vi "Renishaw-XL80_GetExpansionCoefficient.vi"(8 "error in (no error)":errorcluster, 11 "Renishaw-XL80_EMU in":refnum<class "Renishaw-XL80_EMU.lvclass">) -> (0 "error out":errorcluster, 2 "ExpansionCoefficient":dbl, 3 "Renishaw-XL80_EMU out":refnum<class "Renishaw-XL80_EMU.lvclass">)   [LabVIEW 2024, in "Renishaw-XL80_EMU.lvclass"]
doc: "Reading this property retrieves the current material expansion coefficient in ppm/°C.\n\nDefinition\nHRESULTget_ExpansionCoefficient( [out, retval] double* pVal);\nParameters\npVal\nA variable that will be set to the current material expansion coefficient (in ppm/°C).\n\nComments\nReading this property will always retrieve the current material expansion coefficient.\n\nThe property will normally return an HRESULT of S_OK. However, it will return E_POINTER if the client supplies a null pointer for pVal."
uses:
  Renishaw-XL80_EMU.lvclass
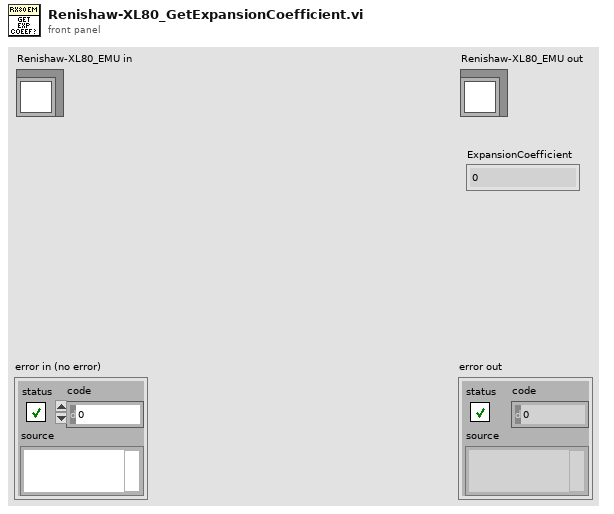
[diagram p1: front panel]
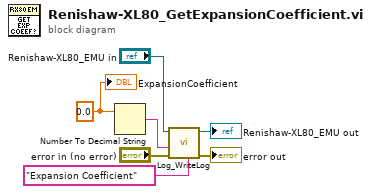
[diagram p0: block diagram]
diagram:
  w2 = 0.0 ("ExpansionCoefficient")
  n1 = Number To Decimal String(number=w2) -> (decimal integer string=w1:string)  [unwired: 1 in]
  n2 = call-dynamic "Log_WriteLog.vi"("Additional text"="Expansion Coefficient", "error in (no error)"="error in (no error)", "Response"=w1, "Log in"="Renishaw-XL80_EMU in") -> ("error out"=→"error out":errorcluster, "Log out"=→"Renishaw-XL80_EMU out":refnum<class "Renishaw-XL80_EMU.lvclass">)  [unwired: 6 in]
  "ExpansionCoefficient" <- w2
